vi "LuaVIEW Swap Task.vi"(0 "script file or name (no name)":path, 5 "custom search directory (none)":path, 7 "script string (\"\" == load from file)":string, 9 "identifier (use keyword)":string, 11 "error in (no error)":errorcluster) -> (8 "identifier":string, 15 "error out":errorcluster)   [LabVIEW 2012]
doc: "Swap the script(s) executing under an existing LuaVIEW task. This VI loads, pre-processes, and compiles the new script(s), and signals the task to be swapped to execute the new script(s). This VI does not wait for the task to commence with swapping: any run-time error that occurs on cleaning up the prior script(s) or on executing the new script(s) is not returned by this VI."
uses:
  typedefs/t_LuaVIEW Task List Methods.ctl
  typedefs/t_LuaVIEW Prepared Script Infos Methods.ctl
  typedefs/t_LuaVIEW Task State Methods.ctl
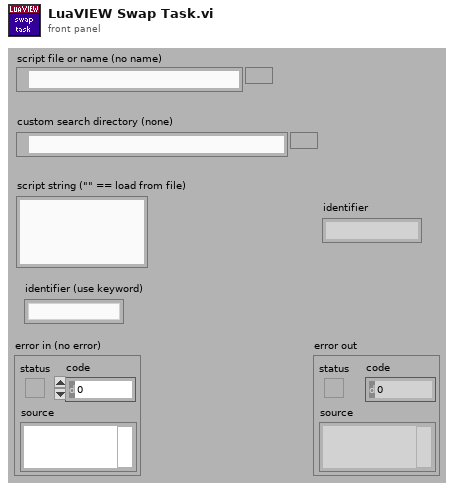
[diagram p1: front panel]
types:
  T1 = typedef "t_LuaVIEW Task List Methods.ctl" = enum16{"clear list", "add", "test", "remove", "get ref", "get task info", "get list", "get script info", "ongoing?", "resume", "pause", "stop", "confirm", "message"}
  T2 = typedef "t_LuaVIEW Prepared Script Infos Methods.ctl" = enum16{"isempty?", "empty", "set", "discard"}
  T3 = typedef "t_LuaVIEW Task State Methods.ctl" = enum16{"cleanup", "set initial", "set mode", "set active mode", "set error", "get task info", "get script info", "set signal", "clear signal", "test handled", "test delegated", "test signal", "handle signal", "delegate signal", "allow signal", "disallow signal", "disallow all", "signals?", "delegated signals?", "protection++", "protection--", "protection=0", "message", "next message", "pop message", "message available?", "force stop", "set swap preps", "apply swap preps"}
  T4 = typedef "t_LuaVIEW Task State Pane.ctl" = refnum<vi>
  T5 = typedef "LuaVIEW Task Info.ctl" = cluster{"main script":string, "identifier":string, "class":string, "description":string, "mode":T6, "handler":string, "LuaVIEW reference":T7, "scripts":i32, "hide":bool, "active":bool, "error msg":string, "defer":bool, "launch":enum16{"asynchronous", "manual", "synchronous"}, "main path valid":bool, "start time":dbl, "swap time":dbl, "task VI":refnum<vi>, "prefsys":enum32{"invalid execution system", "user interface", "standard", "instrument i/o", "data acquisition", "other 1", "other 2", "same as caller"}, "priority":enum32{"invalid priority", "background priority", "normal priority", "above normal priority", "high priority", "time critical priority", "subroutine"}, "signal flags":u32, "allow mask":u32, "handle mask":u32, "disallow manual":bool}
  T6 = typedef "t_LuaVIEW Task Modes.ctl" = enum16{"initializing", "running", "executing", "paused", "error", "swapping"}
  T7 = typedef "t_LuaVIEW Reference.ctl" = refnum<k1>
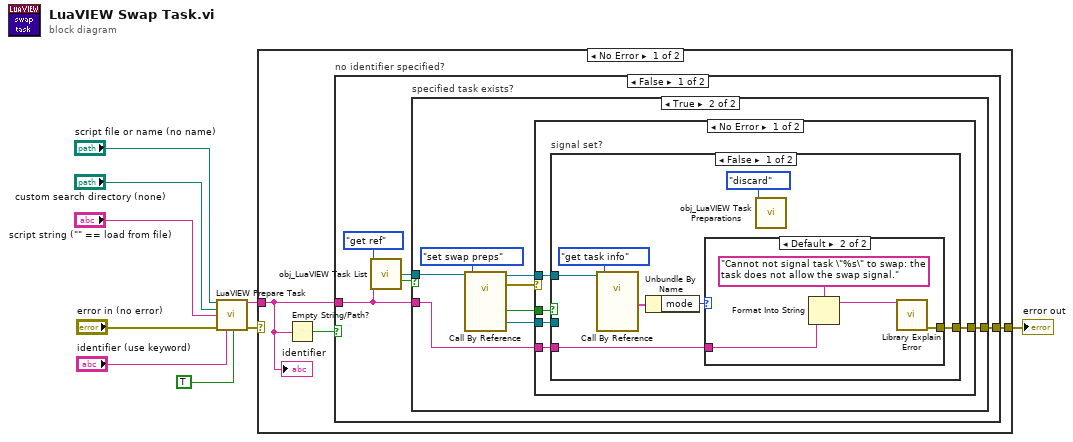
[diagram p0: block diagram]
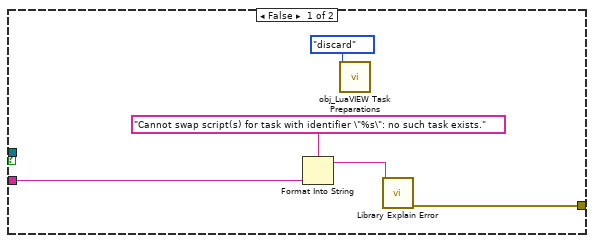
[diagram p2: hidden frame]
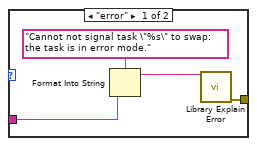
[diagram p3: hidden frame]
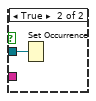
[diagram p4: hidden frame]
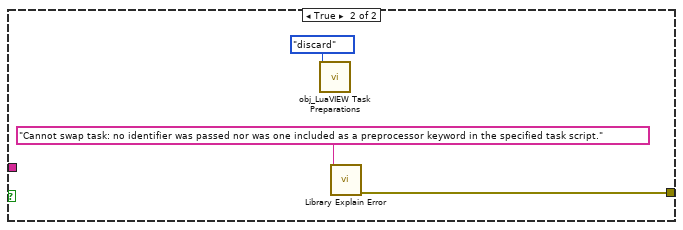
[diagram p6: hidden frame]
diagram:
  n1 = call "LuaVIEW Prepare Task.vi"("script file or name (no name)"="script file or name (no name)", "custom search directory (none)"="custom search directory (none)", "script string (\"\" == load from file)"="script string (\"\" == load from file)", "error in (no error)"="error in (no error)", "identifier (none)"="identifier (use keyword)", "swap? (false)"=TRUE) -> ("identifier"=w2:string, "error out"=w1:errorcluster)  [unwired: 7 in, 1 out]
  n2 = case shown="No Error" w1 {
    selector: w1 -> [_ w56]
    tunnel: [w12 w56] -> w9
    tunnel: w2 -> [w11 _]
    frame No Error {
      n3 = Empty String/Path?(string/path=w11) -> (empty?=w10:bool)
      n4 = case "no identifier specified?" shown="False" w10 {
        tunnel: [w17 w54] -> w12
        tunnel: w11 -> [w13 _]
        frame False {
          n5 = call "obj_LuaVIEW Task List.vi"("method"=t_LuaVIEW_Task_List_Methods."get ref", "task identifier"=w13) -> ("state object ref out"=w15:T4, "set/ongoing"=w14:bool)  [unwired: 8 in, 4 out]
          n6 = case "specified task exists?" shown="True" w14 {
            tunnel: [w19 w30] -> w17
            tunnel: w15 -> [_ w28]
            tunnel: w13 -> [w22 w26]
            frame False {
              n7 = Format Into String(format string="Cannot swap script(s) for task with identifier \"%s\": no such task exists." ("explanation prefix (none)"), w22) -> (resulting string=w20:string)  [unwired: 2 in, 1 out]
              n8 = call "obj_LuaVIEW Task Preparations.vi"("method"=t_LuaVIEW_Prepared_Script_Infos_Methods."discard") -> ()  [unwired: 12 in, 3 out]
              n9 = call "Library Explain Error.vi"("explanation prefix (none)"=w20) -> ("explained error"=w19:errorcluster)  [unwired: 14 in]
            }
            frame True {
              n10 = call-by-ref "?"(reference=w28, "method"=t_LuaVIEW_Task_State_Methods."set swap preps") -> (reference out=w27:T4, error out=w23:errorcluster, "set/available/pending"=w25:bool, "wakeup occurrence"=w24:refnum<k4>)  [unwired: 11 in, 3 out]
              n11 = case shown="No Error" w23 {
                selector: w23 -> [_ w52]
                tunnel: [w35 w52] -> w30
                tunnel: w27 -> [w34 _]
                tunnel: w26 -> [w33 _]
                tunnel: w25 -> [w32 _]
                tunnel: w24 -> [w31 _]
                frame No Error {
                  n12 = case "signal set?" shown="False" w32 {
                    tunnel: [w41 _] -> w35
                    tunnel: w34 -> [w38 _]
                    tunnel: w33 -> [w40 _]
                    tunnel: w31 -> [_ w51]
                    frame False {
                      n13 = call-by-ref "?"(reference=w38, "method"=t_LuaVIEW_Task_State_Methods."get task info") -> ("task info {get task info}"=w37:T5)  [unwired: 11 in, 6 out]
                      n14 = Unbundle By Name(w37) -> ("mode"=w36:T6)
                      n15 = case shown="Default" w36 {
                        tunnel: [w46 w50] -> w41
                        tunnel: w40 -> [w45 w49]
                        frame "error" {
                          n16 = Format Into String(format string="Cannot not signal task \"%s\" to swap: the task is in error mode." ("explanation prefix (none)"), w45) -> (resulting string=w43:string)  [unwired: 2 in, 1 out]
                          n17 = call "Library Explain Error.vi"("explanation prefix (none)"=w43) -> ("explained error"=w46:errorcluster)  [unwired: 14 in]
                        }
                        frame Default {
                          n18 = Format Into String(format string="Cannot not signal task \"%s\" to swap: the task does not allow the swap signal." ("explanation prefix (none)"), w49) -> (resulting string=w47:string)  [unwired: 2 in, 1 out]
                          n19 = call "Library Explain Error.vi"("explanation prefix (none)"=w47) -> ("explained error"=w50:errorcluster)  [unwired: 14 in]
                        }
                      }
                      n20 = call "obj_LuaVIEW Task Preparations.vi"("method"=t_LuaVIEW_Prepared_Script_Infos_Methods."discard") -> ()  [unwired: 12 in, 3 out]
                    }
                    frame True {
                      n21 = Set Occurrence(w51) -> ()
                    }
                  }
                }
                frame Error {
                }
              }
            }
          }
        }
        frame True {
          n22 = call "obj_LuaVIEW Task Preparations.vi"("method"=t_LuaVIEW_Prepared_Script_Infos_Methods."discard") -> ()  [unwired: 12 in, 3 out]
          n23 = call "Library Explain Error.vi"("explanation prefix (none)"="Cannot swap task: no identifier was passed nor was one included as a preprocessor keyword in the specified task script.") -> ("explained error"=w54:errorcluster)  [unwired: 14 in]
        }
      }
      "identifier" <- w11
    }
    frame Error {
    }
  }
  "error out" <- w9
